vi "CLD 17 GUI number pad.vi"() -> ()   [LabVIEW 2009]
doc: "CLD 17\n\nThis VI uses a polling method to respond to changes in the GUI."
uses:
  CLD 17 Keypad_Typedef.ctl
panel:
  out "String":string
  out "Numeric":dbl
  in  "Keypad Cluster":T1
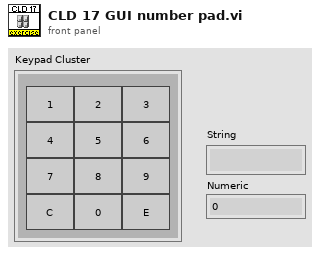
[diagram p1: front panel]
types:
  T1 = typedef "CLD 17 Keypad_Typedef.ctl" = cluster{"0":bool, "1":bool, "2":bool, "3":bool, "4":bool, "5":bool, "6":bool, "7":bool, "8":bool, "9":bool, "C":bool, "E":bool}
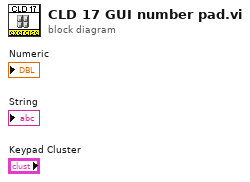
[diagram p0: block diagram]
diagram:
